vi "RF_calibration_NF_WF1974.vi"() -> ()   [LabVIEW 2017]
uses:
  <vilib>/Analysis/6fits.llb/Curve Fitting Criteria.ctl
  instr.lib/Tektronix TDS 200 1000 2000 Series/Tektronix TDS 200 1000 2000 Series.lvlib
  <vilib>/Analysis/NI_AALPro.lvlib
  instr.lib/Keithley 3390/Keithley 3390.lvlib
panel:
  in  "Fit selecter CH1":i32(ring)=1 items=["No fitting", "Linear fit"]
  out "residue CH1":dbl
  out "Fit results CH1 (slope, offset)":dbl[](array[numeric])=[5.825600184872378e+17, 9.899999999999996e+37] format="%_6e"
  out "Graph 2":cluster{dbl[], "Best Linear Fit":dbl[]}[](graph)=[{[10000.0, 20000.0, 30000.0, 40000.0, 50000.0, 60000.0, 70000.0, 80000.0, 90000.0, 100000.0, 110000.0, 120000.0, 130000.0, 140000.0, 150000.0, 160000.0], "Best Linear Fit"=[9.9e+37, 9.9e+37, 9.9e+37, 9.9e+37, 9.9e+37, 9.9e+37, 9.9e+37, 9.9e+37, 9.9e+37, 9.9e+37, 9.9e+37, 9.9e+37, 9.9e+37, 9.9e+37, 9.9e+37, 9.9e+37]}, {[10000.0, 20000.0, 30000.0, 40000.0, 50000.0, 60000.0, 70000.0, 80000.0, 90000.0, 100000.0, 110000.0, 120000.0, 130000.0, 140000.0, 150000.0, 160000.0], "Best Linear Fit"=[9.899999999999996e+37, 9.899999999999997e+37, 9.899999999999997e+37, 9.899999999999997e+37, 9.9e+37, 9.9e+37, 9.9e+37, 9.9e+37, 9.900000000000001e+37, 9.900000000000001e+37, 9.900000000000001e+37, 9.900000000000003e+37, 9.900000000000003e+37, 9.900000000000003e+37, 9.900000000000005e+37, 9.900000000000005e+37]}]
  out "Graph":cluster{dbl[], "Best Linear Fit":dbl[]}[](graph)
  in  "Tab Control":enum32{"CONFIG", "MAIN", "DIAGNOSIS"}(tab)
  in  "WF1974":refnum<visa-resource-name>="USB0::0x0D4A::0x000E::9260521::INSTR"
  in  "Columns":string[](array[string])=["FG freq (Hz)", "FG V (mVpp)", "CH1 Monitor (Vpp)", "CH2 VR (Vpp)"]
  in  "File path":path=path "C:/LabVIEW/DATA/J-PARC_202206/RF"
  in  "Tektronix":refnum<visa-resource-name>="USB0::0x0699::0x0365::C035183::INSTR"
  out "File ref (calibration)":refnum<file>
  in  "COMMENT":string="L1_measurement"
  out "Error Out":errorcluster={"status"=FALSE, "code"=1073676290, "source"="NF WF1973_74 Initialize.vi->RF_calibration_NF_WF1974.vi内のVISAイベント有効"}
  in  "Tektronix test":bool
  in  "Refresh graph":bool
  out "current step":i32=15
  in  "sweep stop":bool=TRUE
  in  "sweep start":bool
  in  "Tab Control 2":T1(tab)
  in  "f_start (Hz)":dbl=10000.0 format="%_8e"
  in  "f_end (Hz)":dbl=200000.0 format="%_8e"
  in  "Δf / cycle (Hz)":dbl=10000.0 format="%_8e"
  in  "V_start (mVamp)":dbl=2000.0 format="%_6f"
  in  "V_end (mVamp)":dbl=8000.0 format="%_6f"
  in  "ΔV / cycle (mVamp)":dbl=500.0 format="%_6f"
  in  "freq/amp":bool
  in  "Vamp lower lim":dbl=0.4 format="%_4f"
  in  "Vamp upper lim":dbl=9000.0 format="%_4f"
  in  "FG reset":bool
  in  "Amplitude (mVpp)":dbl=4000.0 format="%_6f"
  in  "FG Output":bool
  in  "Frequency (Hz)":dbl=160000.0 format="%_8e"
  out "# of steps":i32=19
  out "Measurement index":i32=76
  out "Latest measurement":dbl[](array[numeric])=[160000.0, 4000.0, 0.0824000016, 9.9e+37] format="%_8g"
  out "CH 1 measurement":dbl=0.0824000016 format="%_6g"
  out "CH 2 measurement":dbl=9.9e+37 format="%_6g"
  in  "Fit selecter":i32(ring)=1 items=["No fitting", "Linear fit"]
  out "residue CH2":dbl
  out "Fit results CH2 (slope, offset)":dbl[](array[numeric])=[5.825600184872378e+17, 9.899999999999996e+37] format="%_6e"
  out "error out (Agilent)":errorcluster
  out "error out (Tektronix)":errorcluster={"status"=TRUE, "code"=-1073807240, "source"="Tektronix TDS 200 1000 2000 Series.lvlib:Initialize.vi->RF_calibration_NF_WF1974.vi内のVISAクリア"}
  out "error out (file operation)":errorcluster
  in  "STOP":bool
  # "SWEEP SETTING"
  # "FG CONTROL"
  # "Frequency sweep"
  # "Amplitude sweep"
  # "TEKTRONIX SETTING"
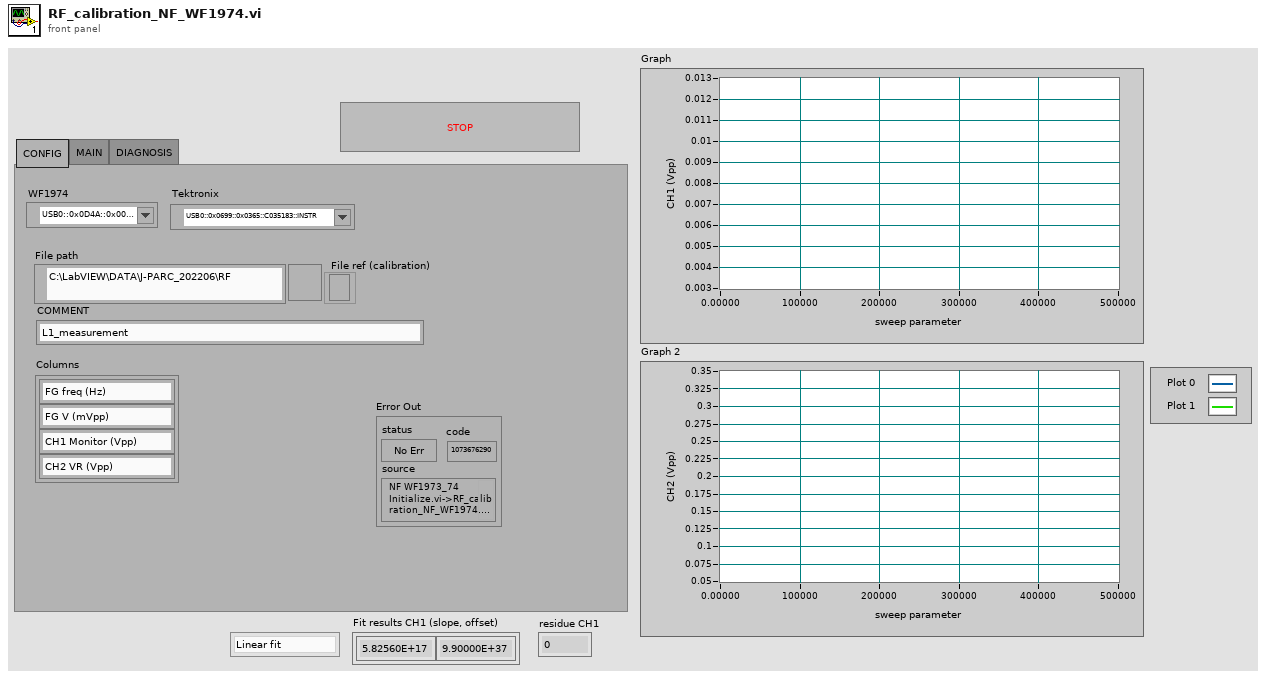
[diagram p1: front panel]
types:
  T1 = enum32{"frequency sweep config", "amplitude sweep config"}
  T2 = cluster{"Baud Rate":u32, "Parity":u16, "Stop Bits":u16, "Flow Control":u16}
  T3 = enum16{"open", "replace", "create", "open or create", "replace or create", "replace or create with confirmation"}
  T4 = cluster{"slope min":dbl, "slope max":dbl, "intercept min":dbl, "intercept max":dbl}
  T5 = cluster{"appended array":dbl[], "appended array":dbl[]}
  T6 = cluster{"appended array":dbl[], "appended array":dbl[]}[]
  T7 = typedef "NI_AALPro.lvlib/Curve Fitting Criteria.ctl" = u16
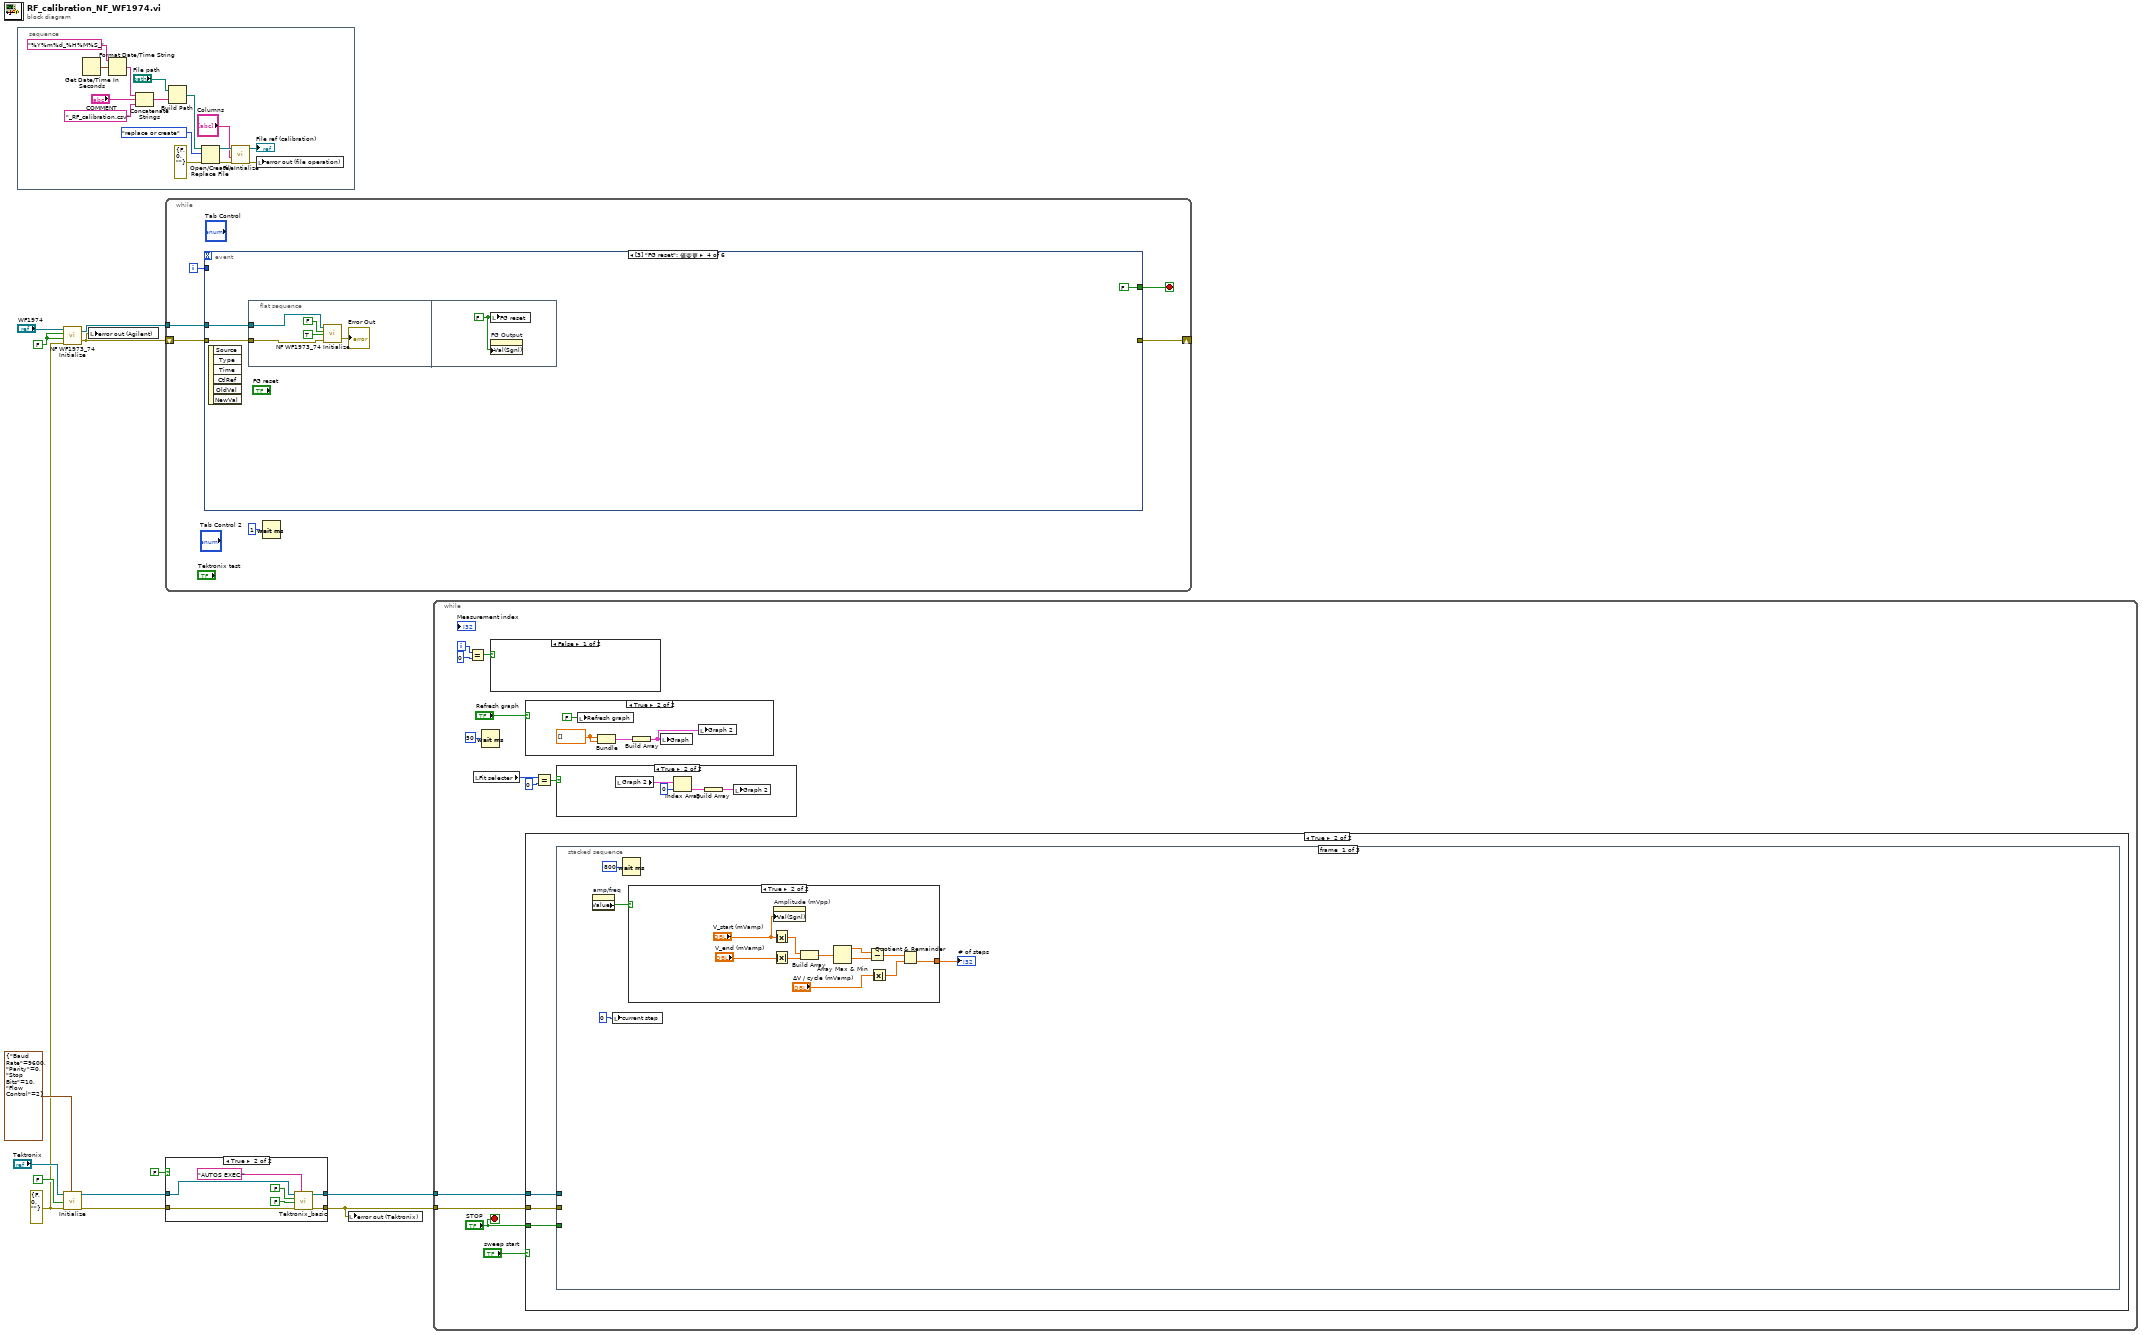
[diagram p0: block diagram]
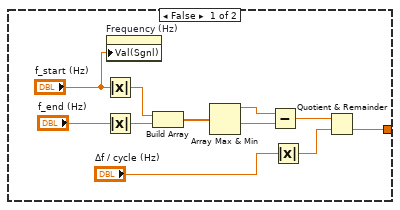
[diagram p6: hidden frame]
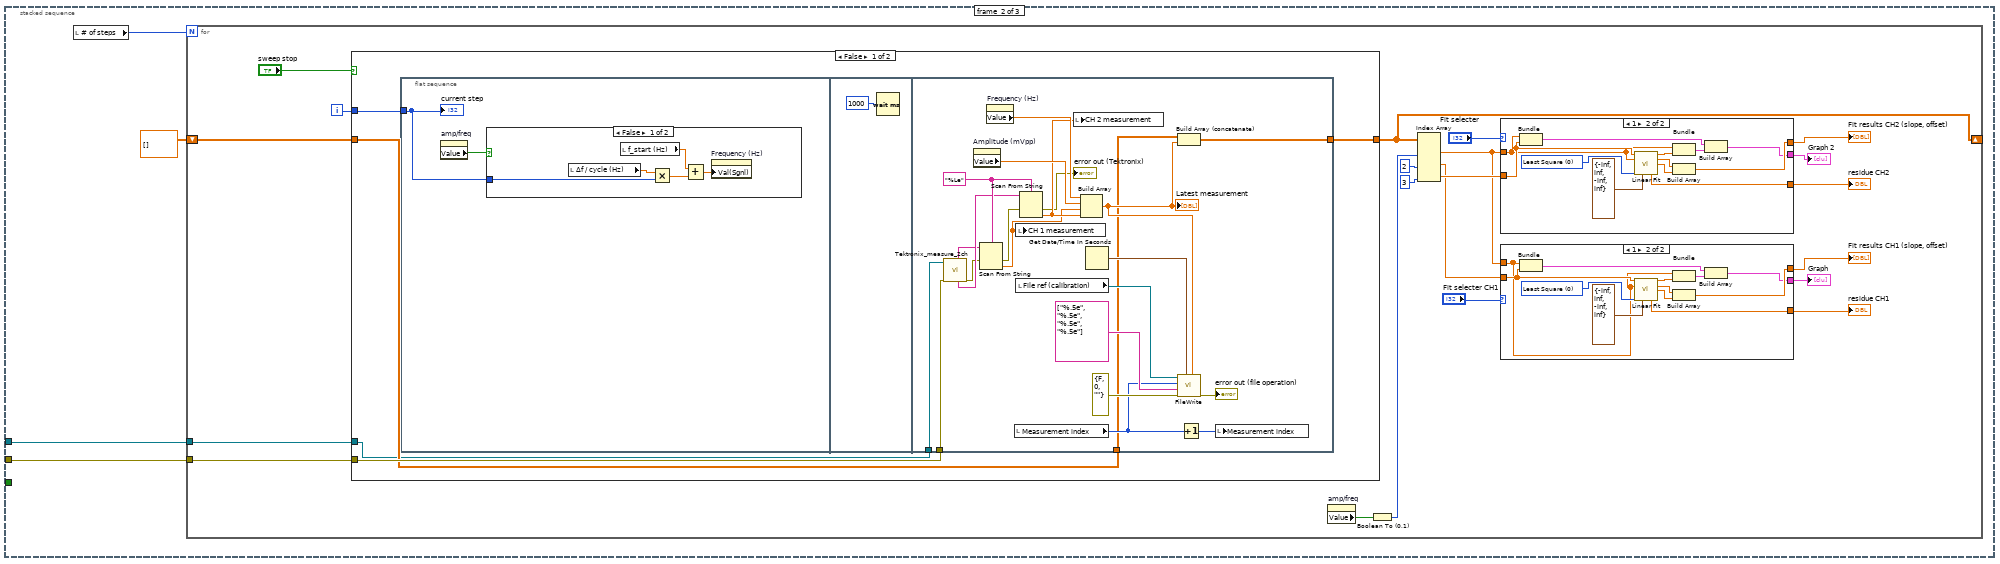
[diagram p7: hidden frame]
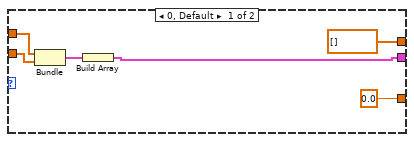
[diagram p8: hidden frame]
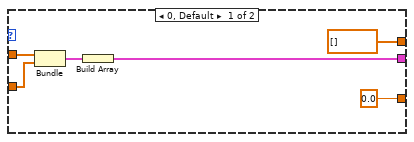
[diagram p9: hidden frame]
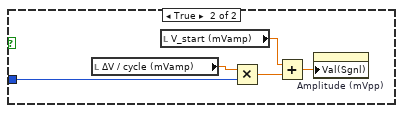
[diagram p10: hidden frame]
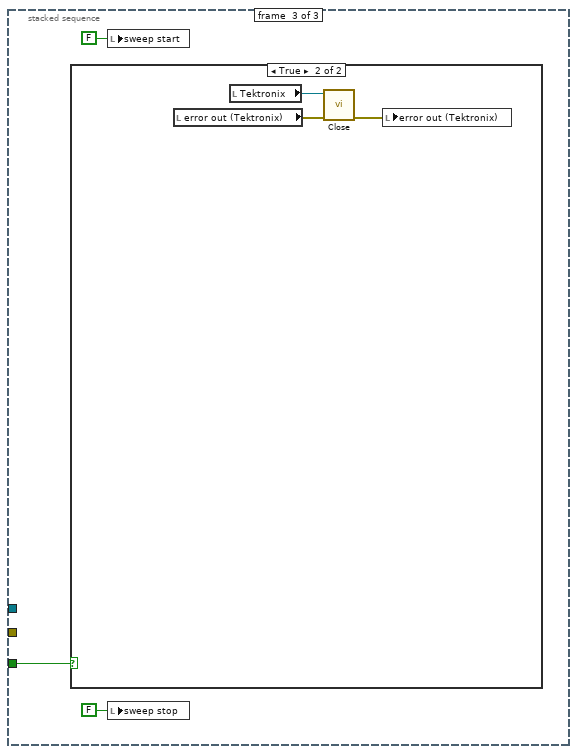
[diagram p12: hidden frame]
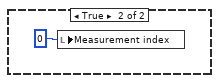
[diagram p14: hidden frame]
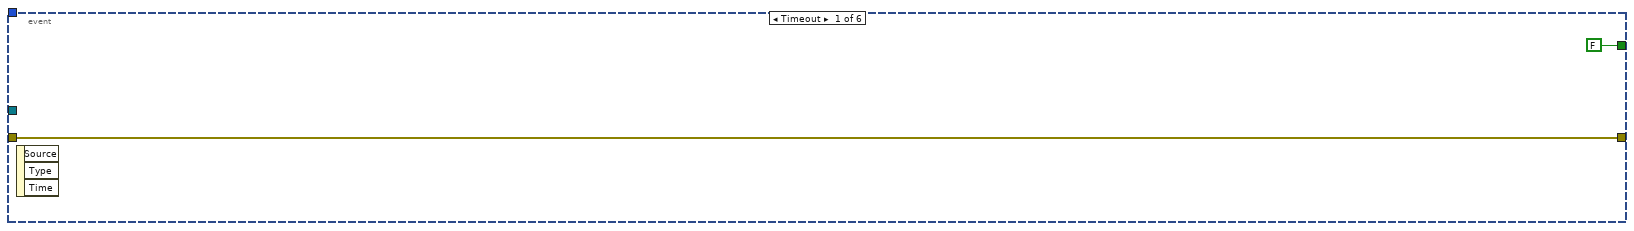
[diagram p15: hidden frame]
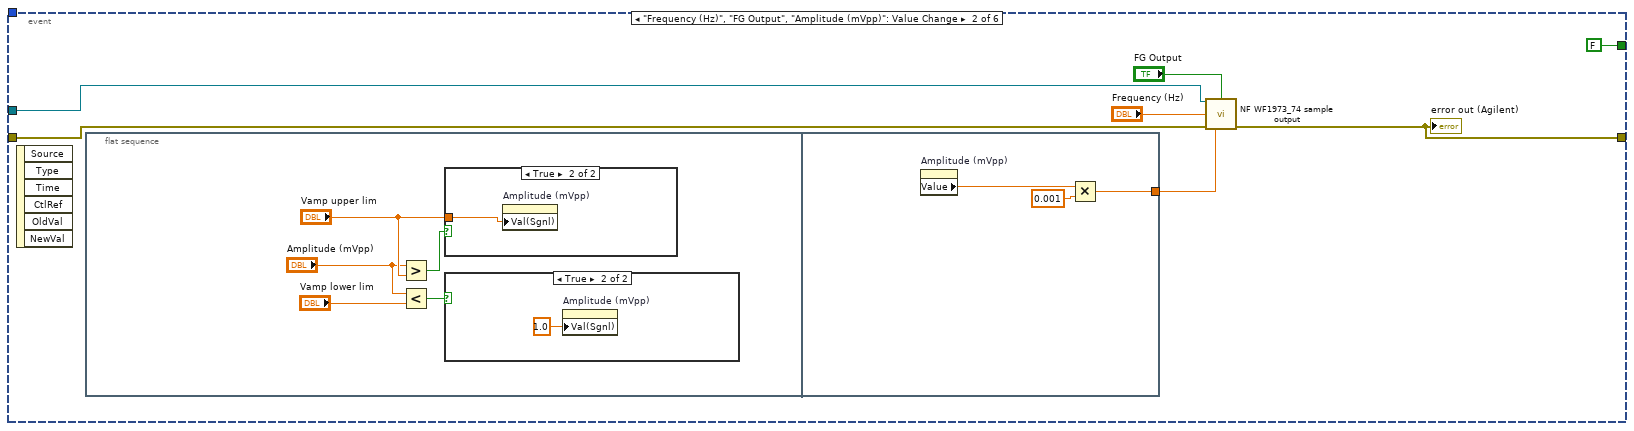
[diagram p16: hidden frame]
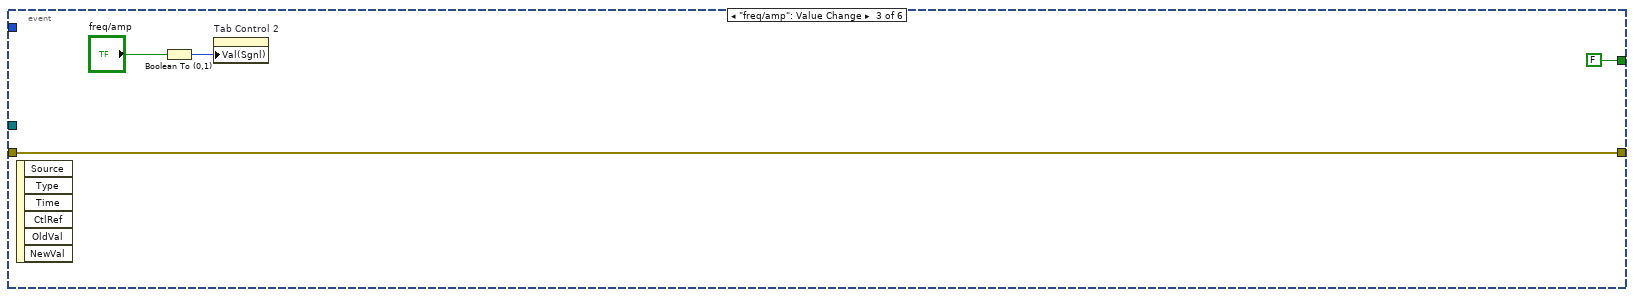
[diagram p19: hidden frame]
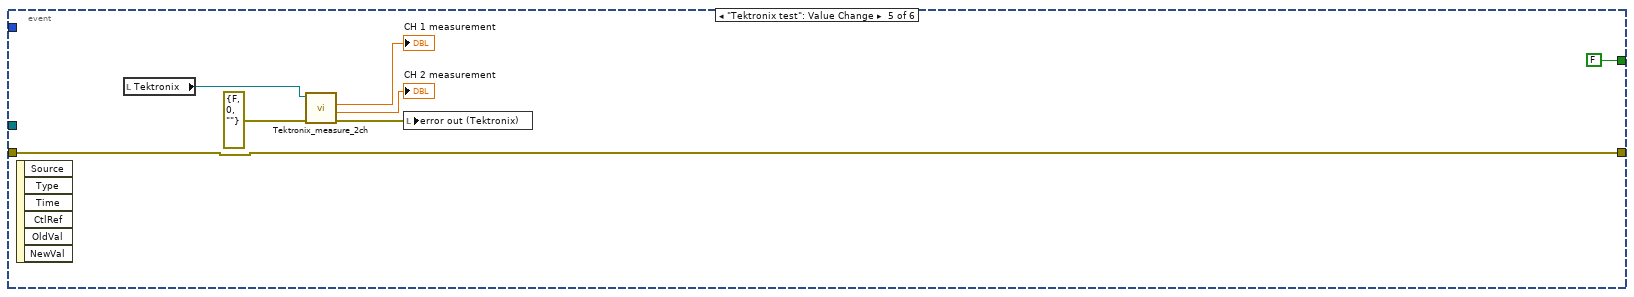
[diagram p20: hidden frame]
diagram:
  w1 = FALSE ("Reset (True)")
  w4 = errorcluster {"status"=FALSE, "code"=0, "source"=""} ("error in (no error)")
  n1 = stacked-sequence {
    frame #0 {
      n2 = Get Date/Time In Seconds() -> (seconds since 1Jan1904=w17:timestamp)
      n3 = Format Date/Time String(time format string (%c)="%Y%m%d_%H%M%S_", seconds (now)=w17) -> (date/time string=w15:string)  [unwired: 1 in]
      n4 = Concatenate Strings(w15, "COMMENT", "_RF_calibration.csv") -> (w28:string)
      n5 = Build Path(base path="File path", name or relative path=w28) -> (appended path=w27:path)
      n6 = Open/Create/Replace File(file path (use dialog)=w27, error in=errorcluster {"status"=FALSE, "code"=0, "source"=""}, operation (0:open)=T3."replace or create") -> (refnum out=w24:refnum<file>, error out=w25:errorcluster)  [unwired: 3 in, 1 out]
      n7 = call "FileIntialize.vi"("Error In"=w25, "Labels"="Columns", "refnum in"=w24) -> ("Error Out"=w14:errorcluster, "File Refnum"=→"File ref (calibration)":refnum<file>)  [unwired: 7 in]
      n8 = local write "error out (file operation)"(w14) -> ()
    }
  }
  n9 = call "NF WF1973_74 Initialize.vi"("Error In"=w4, "Reset(T)"=w1, "ID Check(T)"=w1, "VISAsession"="WF1974") -> ("Error Out"=w3:errorcluster, "CopyVISAsession"=w2:refnum<visa-resource-name>)
  n10 = call "Initialize.vi"("Serial Configuration"=T2 {"Baud Rate"=9600, "Parity"=0, "Stop Bits"=10, "Flow Control"=2}, "error in (no error)"=w4, "Reset? (T: Yes)"=FALSE, "VISA resource name"="Tektronix") -> ("error out"=w10:errorcluster, "VISA resource name out"=w9:refnum<visa-resource-name>)  [unwired: 1 in, 5 out]
  n11 = local write "error out (Agilent)"(w3) -> ()
  n12 = while {
    tunnel: w2 -> [w34]
    shift-right: [w31] -> _
    shift-left: w3 -> [w30]
    i -> [w29]
    stop <- w32 stop-if-true
    n13 = event shown="[3] \"FG reset\": 値変更" {
      selector: _ -> [_ _ _ _ _ _]
      dyn-events: _ -> [_ _ _ _ _ _]
      timeout: _ -> [_ _ _ _ _ _]
      tunnel: w34 -> [_ w42 _ w59 _ w79]
      tunnel: w30 -> [w35 w41 w55 w58 w68 w75]
      tunnel: [FALSE FALSE FALSE FALSE FALSE TRUE] -> w32
      tunnel: [w35 w37 w55 _ w68 w74] -> w31
      tunnel: w29 -> [_ _ _ _ _ _]
      event Timeout {
        n14 = event-data() -> ()  [unwired: 1 in, 3 out]
      }
      event "Frequency (Hz)", "FG Output", "Amplitude (mVpp)": Value Change {
        n15 = event-data() -> ()  [unwired: 1 in, 6 out]
        n16 = flat-sequence {
          tunnel: [w52] -> w38
          frame #0 {
            n17 = Greater?(x="Amplitude (mVpp)", y="Vamp upper lim") -> (0:w47:bool)
            n18 = Less?(x="Amplitude (mVpp)", y="Vamp lower lim") -> (x < y?=w44:bool)
            n19 = case shown="TRUE" w47 {
              tunnel: "Vamp upper lim" -> [_ w50]
              frame False {
              }
              frame True {
                n20 = property on="Amplitude (mVpp)" class="DigNum （指定）"("Val(Sgnl)"=w50) -> ()  [unwired: 2 in, 2 out]
              }
            }
            n21 = case shown="TRUE" w44 {
              frame False {
              }
              frame True {
                n22 = property on="Amplitude (mVpp)" class="DigNum （指定）"("Val(Sgnl)"=1.0 ("Value (Signaling)")) -> ()  [unwired: 2 in, 2 out]
              }
            }
          }
          frame #1 {
            n23 = property on="Amplitude (mVpp)" class="DigNum （指定）"() -> ("Value"=w51:dbl)  [unwired: 2 in, 2 out]
            n24 = Multiply(x=w51, y=0.001) -> (x*y=w52:dbl)
          }
        }
        n25 = call "NF WF1973_74 sample output.vi"("VISAsession"=w42, "OUTPUT?(OFF)"="FG Output", "Frequency(1)"="Frequency (Hz)", "error in (no error)"=w41, "Amplitude(1)"=w38) -> ("error out"=w37:errorcluster)  [unwired: 9 in, 1 out]
        "error out (Agilent)" <- w37
      }
      event "freq/amp": Value Change {
        n26 = event-data() -> ()  [unwired: 1 in, 6 out]
        n27 = Boolean To (0,1)(Boolean="freq/amp") -> (0, 1=w56:i16)
        n28 = property on="Tab Control 2" class="TabCtl （指定）"("Val(Sgnl)"=w56) -> ()  [unwired: 2 in, 2 out]
      }
      event "FG reset": Value Change {
        n29 = event-data() -> ()  [unwired: 1 in, 6 out]
        n30 = flat-sequence {
          tunnel: w58 -> [w62]
          tunnel: w59 -> [w65]
          frame #0 {
            n31 = call "NF WF1973_74 Initialize.vi"("Error In"=w62, "Reset(T)"=TRUE, "ID Check(T)"=FALSE ("ID Query (True)"), "VISAsession"=w65) -> ("Error Out"=→"Error Out":errorcluster)  [unwired: 1 out]
          }
          frame #1 {
            w66 = FALSE ("Value (Signaling)")
            n32 = local write "FG reset"(w66) -> ()
            n33 = property on="FG Output" class="Bool （指定）"("Val(Sgnl)"=w66) -> ()  [unwired: 2 in, 2 out]
          }
        }
      }
      event "Tektronix test": Value Change {
        n34 = event-data() -> ()  [unwired: 1 in, 6 out]
        n35 = local read "Tektronix"() -> (w73:refnum<visa-resource-name>)
        n36 = call "Tektronix_measure_2ch.vi"("error in (no error)"=errorcluster {"status"=FALSE, "code"=0, "source"=""}, "VISA resource name"=w73) -> ("error out"=w69:errorcluster, "Measurement 2"=→"CH 2 measurement":dbl, "Measurement 1"=→"CH 1 measurement":dbl)  [unwired: 4 in, 3 out]
        n37 = local write "error out (Tektronix)"(w69) -> ()
      }
      event "STOP": Value Change {
        w77 = FALSE ("Enable Output  (T: Enable)")
        n38 = event-data() -> ()  [unwired: 1 in, 6 out]
        n39 = property on="FG Output" class="Bool （指定）"("Val(Sgnl)"=w77) -> ()  [unwired: 2 in, 2 out]
        n40 = call "Enable Output.vi"("Enable Output (T: Enable)"=w77, "error in (no error)"=w75, "VISA resource name"=w79) -> ("error out"=w78:errorcluster, "VISA resource name out"=w80:refnum<visa-resource-name>)  [unwired: 7 in]
        n41 = call "Close.vi"("error in (no error)"=w78, "VISA resource name"=w80) -> ("error out"=w74:errorcluster)  [unwired: 9 in]
        n42 = local write "error out (Agilent)"(w74) -> ()
      }
    }
    n43 = Wait (ms)(milliseconds to wait=u32 1) -> ()  [unwired: 1 out]
  }
  n44 = case shown="TRUE" FALSE {
    tunnel: w10 -> [w81 w89]
    tunnel: w9 -> [w82 w88]
    tunnel: [w82 w87] -> w8
    tunnel: [w81 w86] -> w7
    frame False {
    }
    frame True {
      n45 = call "Tektronix_basic.vi"("write buffer"="AUTOS EXEC;", "error in (no error)"=w89, "Query?"=FALSE, "Error query?"=FALSE, "VISA resource name"=w88) -> ("error out"=w86:errorcluster, "VISA resource name out"=w87:refnum<visa-resource-name>)  [unwired: 4 in, 1 out]
    }
  }
  n46 = local write "error out (Tektronix)"(w7) -> ()
  n47 = while {
    tunnel: w7 -> [w96]
    tunnel: w8 -> [w93]
    i -> [w101]
    stop <- "STOP" stop-if-true
    n48 = Equal?(x=w101, y=0) -> (x = y?=w99:bool)
    n49 = local read "Fit selecter"() -> (w92:i32)
    n50 = Wait (ms)(milliseconds to wait=u32 50) -> ()  [unwired: 1 out]
    n51 = case shown="FALSE" w99 {
      frame False {
      }
      frame True {
        n52 = local write "Measurement index"(0 ("Measurement index")) -> ()
      }
    }
    n53 = case shown="TRUE" "Refresh graph" {
      frame False {
      }
      frame True {
        w109 = dbl[] [] ("appended array")
        n54 = local write "Refresh graph"(FALSE ("Refresh graph")) -> ()
        n55 = Bundle("appended array"=w109, "appended array"=w109) -> (w107:T5)  [unwired: 1 in]
        n56 = Build Array(w107) -> (w106:T6)
        n57 = local write "Graph"(w106) -> ()
        n58 = local write "Graph 2"(w106) -> ()
      }
    }
    n59 = case shown="TRUE" "sweep start" {
      tunnel: w96 -> [_ w112]
      tunnel: "STOP" -> [_ w111]
      tunnel: w93 -> [_ w110]
      frame False {
      }
      frame True {
        n60 = stacked-sequence {
          tunnel: w112 -> [_ w142 _]
          tunnel: w111 -> [_ _ w243]
          tunnel: w110 -> [_ w139 _]
          frame #0 {
            n61 = property on="amp/freq" class="Bool （指定）"() -> ("Value"=w115:bool)  [unwired: 2 in, 2 out]
            n62 = local write "current step"(0 ("current step")) -> ()
            n63 = Wait (ms)(milliseconds to wait=u32 800) -> ()  [unwired: 1 out]
            n64 = case shown="TRUE" w115 {
              tunnel: [w117 w128] -> w116
              frame False {
                n65 = Absolute Value(x="f_start (Hz)") -> (abs(x)=w124:dbl)
                n66 = Absolute Value(x="f_end (Hz)") -> (abs(x)=w123:dbl)
                n67 = property on="Frequency (Hz)" class="DigNum （指定）"("Val(Sgnl)"="f_start (Hz)") -> ()  [unwired: 2 in, 2 out]
                n68 = Build Array(w124, w123) -> (w122:dbl[])
                n69 = Array Max & Min(array=w122) -> (max value=w121:dbl, min value=w120:dbl)  [unwired: 2 out]
                n70 = Subtract(x=w121, y=w120) -> (x-y=w119:dbl)
                n71 = Absolute Value(x="Δf / cycle (Hz)") -> (abs(x)=w126:dbl)
                n72 = Quotient & Remainder(x=w119, y=w126) -> (floor(x/y)=w117:dbl)  [unwired: 1 out]
              }
              frame True {
                n73 = Absolute Value(x="V_start (mVamp)") -> (abs(x)=w131:dbl)
                n74 = Absolute Value(x="V_end (mVamp)") -> (abs(x)=w132:dbl)
                n75 = property on="Amplitude (mVpp)" class="DigNum （指定）"("Val(Sgnl)"="V_start (mVamp)") -> ()  [unwired: 2 in, 2 out]
                n76 = Build Array(w131, w132) -> (w133:dbl[])
                n77 = Array Max & Min(array=w133) -> (max value=w134:dbl, min value=w135:dbl)  [unwired: 2 out]
                n78 = Subtract(x=w134, y=w135) -> (x-y=w136:dbl)
                n79 = Absolute Value(x="ΔV / cycle (mVamp)") -> (abs(x)=w138:dbl)
                n80 = Quotient & Remainder(x=w136, y=w138) -> (floor(x/y)=w128:dbl)  [unwired: 1 out]
              }
            }
            "# of steps" <- w116
          }
          frame #1 {
            n81 = local read "# of steps"() -> (w141:i32)
            n82 = for {
              N: w141 -> [_]
              tunnel: w142 -> [w162]
              shift-right: [w159] -> _
              shift-left: dbl[][] [] -> [w160]
              tunnel: w139 -> [w154]
              i -> [w163]
              n83 = case shown="FALSE" "sweep stop" {
                tunnel: w163 -> [w204 _]
                tunnel: w162 -> [w203 _]
                tunnel: [w202 w240] -> w159
                tunnel: w160 -> [w201 w240]
                tunnel: w154 -> [w200 _]
                frame False {
                  n84 = flat-sequence {
                    tunnel: w204 -> [w205]
                    tunnel: w203 -> [w236]
                    tunnel: [w229] -> w202
                    tunnel: w201 -> [w227]
                    tunnel: w200 -> [w226]
                    frame #0 {
                      n85 = property on="amp/freq" class="Bool （指定）"() -> ("Value"=w206:bool)  [unwired: 2 in, 2 out]
                      n86 = case shown="FALSE" w206 {
                        tunnel: w205 -> [w209 w214]
                        frame False {
                          n87 = local read "Δf / cycle (Hz)"() -> (w210:dbl)
                          n88 = local read "f_start (Hz)"() -> (w211:dbl)
                          n89 = Multiply(x=w210, y=w209) -> (x*y=w208:dbl)
                          n90 = Add(x=w211, y=w208) -> (x+y=w207:dbl)
                          n91 = property on="Frequency (Hz)" class="DigNum （指定）"("Val(Sgnl)"=w207) -> ()  [unwired: 2 in, 2 out]
                        }
                        frame True {
                          n92 = local read "ΔV / cycle (mVamp)"() -> (w215:dbl)
                          n93 = local read "V_start (mVamp)"() -> (w216:dbl)
                          n94 = Multiply(x=w215, y=w214) -> (x*y=w213:dbl)
                          n95 = Add(x=w216, y=w213) -> (x+y=w212:dbl)
                          n96 = property on="Amplitude (mVpp)" class="DigNum （指定）"("Val(Sgnl)"=w212) -> ()  [unwired: 2 in, 2 out]
                        }
                      }
                      "current step" <- w205
                    }
                    frame #1 {
                      n97 = Wait (ms)(milliseconds to wait=u32 1000) -> ()  [unwired: 1 out]
                    }
                    frame #2 {
                      w223 = "%Le" ("format string")
                      n98 = call "Tektronix_measure_2ch.vi"("error in (no error)"=w236, "VISA resource name"=w226) -> ("error out"=w219:errorcluster, "read buffer 2"=w222:string, "read buffer 1"=w221:string)  [unwired: 4 in, 3 out]
                      n99 = property on="Amplitude (mVpp)" class="DigNum （指定）"() -> ("Value"=w232:dbl)  [unwired: 2 in, 2 out]
                      n100 = Scan From String(format string=w223, input string=w221, error in=w219) -> (error out=w224:errorcluster, output 1=w220:dbl)  [unwired: 1 in, 3 out]
                      n101 = property on="Frequency (Hz)" class="DigNum （指定）"() -> ("Value"=w233:dbl)  [unwired: 2 in, 2 out]
                      n102 = local read "Measurement index"() -> (w230:i32)
                      n103 = local write "CH 1 measurement"(w220) -> ()
                      n104 = local read "File ref (calibration)"() -> (w239:refnum<file>)
                      n105 = Scan From String(format string=w223, input string=w222, error in=w224) -> (error out=→"error out (Tektronix)":errorcluster, output 1=w225:dbl)  [unwired: 1 in, 3 out]
                      n106 = local write "CH 2 measurement"(w225) -> ()
                      n107 = Build Array(w233, w232, w220, w225) -> (w228:dbl[])
                      "Latest measurement" <- w228
                      n108 = Get Date/Time In Seconds() -> (seconds since 1Jan1904=w235:timestamp)
                      n109 = Build Array (concatenate)(w227, w228) -> (w229:dbl[][])
                      n110 = call "FileWrite.vi"("DataArray"=w228, "Time Stamp"=w235, "Error In"=errorcluster {"status"=FALSE, "code"=0, "source"=""}, "FileFormat"=string[] ["%.5e", "%.5e", "%.5e", "%.5e"], "Index"=w230, "refnum in"=w239) -> ("Error Out"=→"error out (file operation)":errorcluster)  [unwired: 4 in, 1 out]
                      n111 = Increment(x=w230) -> (x+1=w231:i32)
                      n112 = local write "Measurement index"(w231) -> ()
                    }
                  }
                }
                frame True {
                }
              }
              n113 = property on="amp/freq" class="Bool （指定）"() -> ("Value"=w155:bool)  [unwired: 2 in, 2 out]
              n114 = Boolean To (0,1)(Boolean=w155) -> (0, 1=w158:i16)
              n115 = Index Array(array=w159, index (col) #1=w158, index (col) #2=2 ("disabled index (col)"), index (col) #3=3 ("index (row)")) -> (element #1=w144:dbl[], element #2=w143:dbl[], element #3=w148:dbl[])  [unwired: 3 in]
              n116 = case shown="1" "Fit selecter" {
                tunnel: w148 -> [w184 w192]
                tunnel: [0.0 ("residue") w195] -> w152
                tunnel: [dbl[] [] w194] -> w151
                tunnel: w144 -> [w185 w191]
                tunnel: [w182 w188] -> w150
                frame 0, Default {
                  n117 = Bundle(w185, w184) -> (w183:cluster{dbl[], dbl[]})  [unwired: 1 in]
                  n118 = Build Array(w183) -> (w182:cluster{dbl[], dbl[]}[])
                }
                frame 1 {
                  w199 = T7 0 items=["Least Square", "Least Absolute Residual", "Bisquare"] ("method")
                  n119 = Bundle(w191, w192) -> (w190:cluster{dbl[], dbl[]})  [unwired: 1 in]
                  n120 = call <vilib>:"Linear Fit.vi"("Y"=w192, "X"=w191, "method"=w199, "parameter bounds"=T4 {"slope min"=-inf, "slope max"=inf, "intercept min"=-inf, "intercept max"=inf}) -> ("Best Linear Fit"=w193:dbl[], "slope"=w197:dbl, "intercept"=w196:dbl, "residue"=w195:dbl)  [unwired: 7 in, 1 out]
                  n121 = Bundle(w191, "Best Linear Fit"=w193) -> (w189:cluster{dbl[], "Best Linear Fit":dbl[]})  [unwired: 1 in]
                  n122 = Build Array(w197, w196) -> (w194:dbl[])
                  n123 = Build Array(w190, w189) -> (w188:cluster{dbl[], "Best Linear Fit":dbl[]}[])
                }
              }
              "Graph 2" <- w150
              "residue CH2" <- w152
              "Fit results CH2 (slope, offset)" <- w151
              n124 = case shown="1" "Fit selecter CH1" {
                tunnel: [0.0 ("residue") w177] -> w145
                tunnel: [dbl[] [] w176] -> w146
                tunnel: w143 -> [w165 w171]
                tunnel: [w164 w173] -> w147
                tunnel: w144 -> [w166 w170]
                frame 0, Default {
                  n125 = Bundle(w166, w165) -> (w167:cluster{dbl[], dbl[]})  [unwired: 1 in]
                  n126 = Build Array(w167) -> (w164:cluster{dbl[], dbl[]}[])
                }
                frame 1 {
                  w181 = T7 0 items=["Least Square", "Least Absolute Residual", "Bisquare"] ("method")
                  n127 = Bundle(w170, w171) -> (w172:cluster{dbl[], dbl[]})  [unwired: 1 in]
                  n128 = call <vilib>:"Linear Fit.vi"("Y"=w171, "X"=w170, "method"=w181, "parameter bounds"=T4 {"slope min"=-inf, "slope max"=inf, "intercept min"=-inf, "intercept max"=inf}) -> ("Best Linear Fit"=w175:dbl[], "slope"=w179:dbl, "intercept"=w178:dbl, "residue"=w177:dbl)  [unwired: 7 in, 1 out]
                  n129 = Bundle(w170, "Best Linear Fit"=w175) -> (w174:cluster{dbl[], "Best Linear Fit":dbl[]})  [unwired: 1 in]
                  n130 = Build Array(w179, w178) -> (w176:dbl[])
                  n131 = Build Array(w172, w174) -> (w173:cluster{dbl[], "Best Linear Fit":dbl[]}[])
                }
              }
              "Graph" <- w147
              "Fit results CH1 (slope, offset)" <- w146
              "residue CH1" <- w145
            }
          }
          frame #2 {
            n132 = case shown="TRUE" w243 {
              frame False {
              }
              frame True {
                n133 = local read "error out (Tektronix)"() -> (w245:errorcluster)
                n134 = local read "Tektronix"() -> (w246:refnum<visa-resource-name>)
                n135 = call "Close.vi"("error in (no error)"=w245, "VISA resource name"=w246) -> ("error out"=w244:errorcluster)  [unwired: 9 out]
                n136 = local write "error out (Tektronix)"(w244) -> ()
              }
            }
            n137 = local write "sweep start"(FALSE ("sweep start")) -> ()
            n138 = local write "sweep stop"(FALSE ("sweep stop")) -> ()
          }
        }
      }
    }
    n139 = Equal?(x=w92, y=0) -> (x = y?=w90:bool)
    n140 = case shown="TRUE" w90 {
      frame False {
      }
      frame True {
        n141 = local read "Graph 2"() -> (w105:cluster{dbl[], "Best Linear Fit":dbl[]}[])
        n142 = Index Array(array=w105, index=0) -> (element=w103:cluster{dbl[], "Best Linear Fit":dbl[]})
        n143 = Build Array(w103) -> (w102:cluster{dbl[], "Best Linear Fit":dbl[]}[])
        n144 = local write "Graph 2"(w102) -> ()
      }
    }
  }
